vi "Simple Traffic Light System( 3 LED ).vi"() -> ()   [LabVIEW 2021]
panel:
  in  "stop":bool
  out "Green":bool
  out "Yellow":bool
  out "Red":bool=TRUE
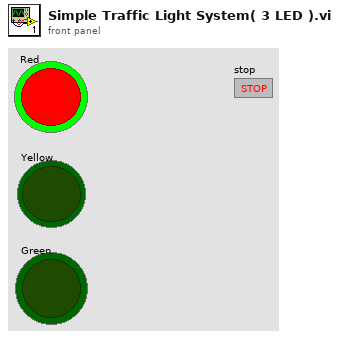
[diagram p1: front panel]
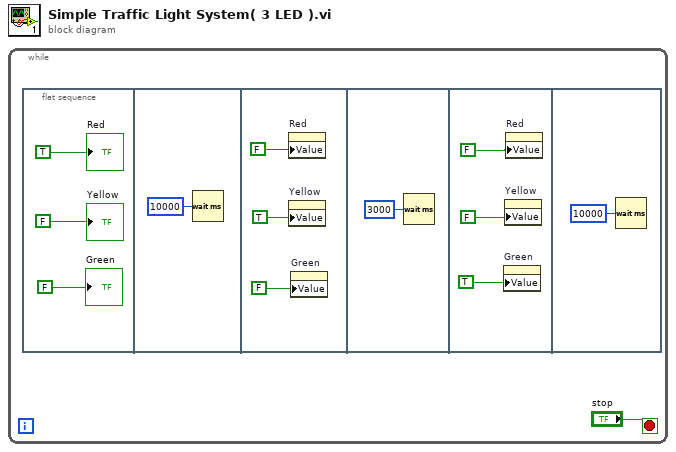
[diagram p0: block diagram]
diagram:
  n1 = while {
    stop <- "stop" stop-if-true
    n2 = flat-sequence {
      frame #0 {
        "Red" <- TRUE
        "Yellow" <- FALSE
        "Green" <- FALSE
      }
      frame #1 {
        n3 = Wait (ms)(milliseconds to wait=u32 10000) -> ()  [unwired: 1 out]
      }
      frame #2 {
        n4 = property on="Red" class="Bool (strict)"("Value"=FALSE) -> ()  [unwired: 2 in, 2 out]
        n5 = property on="Yellow" class="Bool (strict)"("Value"=TRUE) -> ()  [unwired: 2 in, 2 out]
        n6 = property on="Green" class="Bool (strict)"("Value"=FALSE) -> ()  [unwired: 2 in, 2 out]
      }
      frame #3 {
        n7 = Wait (ms)(milliseconds to wait=u32 3000) -> ()  [unwired: 1 out]
      }
      frame #4 {
        n8 = property on="Green" class="Bool (strict)"("Value"=TRUE) -> ()  [unwired: 2 in, 2 out]
        n9 = property on="Yellow" class="Bool (strict)"("Value"=FALSE) -> ()  [unwired: 2 in, 2 out]
        n10 = property on="Red" class="Bool (strict)"("Value"=FALSE) -> ()  [unwired: 2 in, 2 out]
      }
      frame #5 {
        n11 = Wait (ms)(milliseconds to wait=u32 10000) -> ()  [unwired: 1 out]
      }
    }
  }
